vi "XY Graph Compute Interpolated Plot.vi"(8 "Error In":errorcluster, 9 "Ramp":dbl[](array[numeric]), 11 "Plot":T1) -> (0 "Error Out":errorcluster, 3 "Interpolated Plot":T1)   [LabVIEW 2021, in "XY Graph Add-Ons.lvlib"]
uses:
  XY Graph Add-Ons.lvlib
  XY Plot Data.ctl
  <vilib>/Utility/error.llb/Error Cluster From Error Code.vi
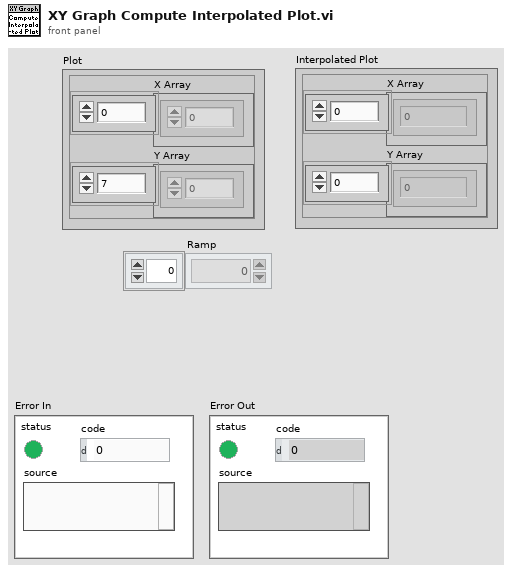
[diagram p1: front panel]
types:
  T1 = typedef "XY Graph Add-Ons.lvlib/XY Plot Data.ctl" = cluster{"X Array":dbl[], "Y Array":dbl[]}
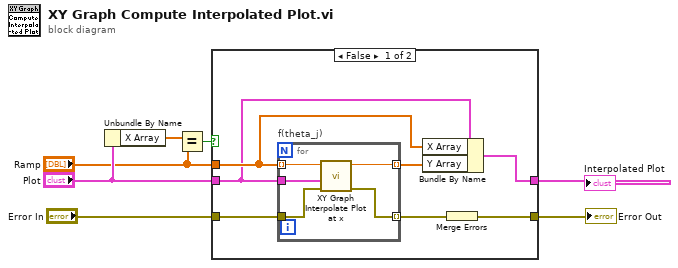
[diagram p0: block diagram]
diagram:
  n1 = Unbundle By Name("Plot") -> ("X Array"=w5:dbl[])
  n2 = Equal?(x=w5, y="Ramp") -> (x = y?=w4:bool)
  n3 = case shown="False" w4 {
    tunnel: "Error In" -> [w14 w20]
    tunnel: [w13 w20] -> w6
    tunnel: "Plot" -> [w10 w21]
    tunnel: "Ramp" -> [w11 _]
    tunnel: [w12 w21] -> w1
    frame False {
      n4 = for "f(theta_j)" {
        tunnel: w10 -> [w19]
        tunnel: w11 -> [w18] mode=indexing
        tunnel: w14 -> [w17]
        tunnel: [w16] -> w8 mode=indexing
        tunnel: [w15] -> w9 mode=indexing
        n5 = call "XY Graph Interpolate Plot at x.vi"("Error In"=w17, "XY Plot"=w19, "t"=w18) -> ("Error Out"=w15:errorcluster, "XY Plot(t)"=w16:dbl)  [unwired: 7 in]
      }
      n6 = Bundle By Name(cluster=w10, "X Array"=w11, "Y Array"=w8) -> (w12:T1)
      n7 = Merge Errors(w9) -> (w13:errorcluster)
    }
    frame True {
      # "No need to interpolate"
    }
  }
  "Error Out" <- w6
  "Interpolated Plot" <- w1
